vi "Generate New Filename.vi"(8 "Filename Suffix (_data.csv)":string="_data.csv", 9 "Time Format String\n(%y_%m_%d__%H_%M_%S%4u)":string="%y_%m_%d__%H_%M_%S%4u", 10 "Output Directory":path=path "C:/Users/Josh/Desktop/code/CVB/Config/generated_data", 11 "Create New File":bool) -> (3 "Output Filename":path)   [LabVIEW 2021]
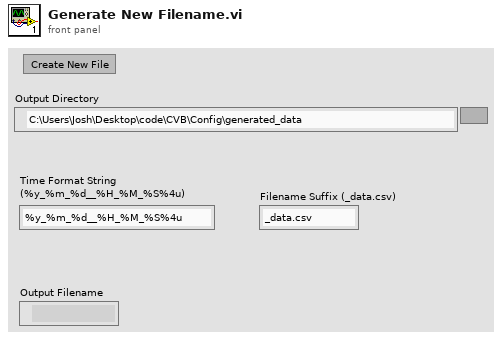
[diagram p1: front panel]
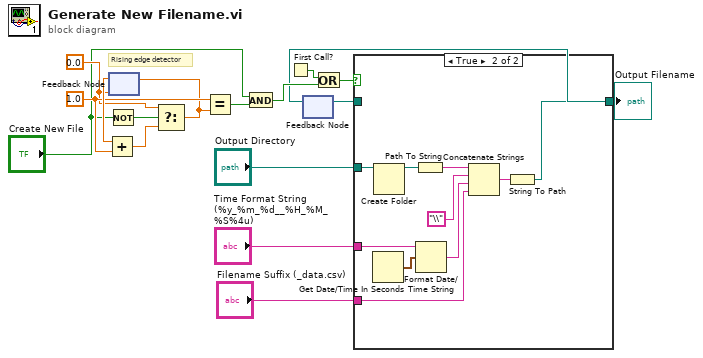
[diagram p0: block diagram]
diagram:
  w12 = 0.0
  w15 = 1.0 ("y")
  # "Rising edge detector"
  n1 = Not(x="Create New File") -> (.not. x?=w10:bool)
  n2 = feedback #1(w12) -> (w16:dbl)
  n3 = Add(x=w16, y=w15) -> (x+y=w11:dbl)
  n4 = Select(t=w12, s=w10, f=w11) -> (s? t:f=w13:dbl)
  n5 = feedback-in #1(w13) -> ()
  n6 = Equal?(x=w15, y=w13) -> (x = y?=w14:bool)
  n7 = And(x="Create New File", y=w14) -> (x .and. y?=w8:bool)
  n8 = First Call?() -> (First Call?: T/F=w7:bool)
  n9 = feedback #2() -> (w6:path)  [unwired: 1 in]
  n10 = Or(x=w7, y=w8) -> (x .or. y?=w9:bool)
  n11 = case shown="True" w9 {
    tunnel: [w17 w20] -> w5
    tunnel: w6 -> [w17 _]
    tunnel: "Output Directory" -> [_ w19]
    tunnel: "Time Format String\n(%y_%m_%d__%H_%M_%S%4u)" -> [_ w22]
    tunnel: "Filename Suffix (_data.csv)" -> [_ w21]
    frame False {
    }
    frame True {
      n12 = Get Date/Time In Seconds() -> (seconds since 1Jan1904=w23:timestamp)
      n13 = Create Folder(path (use dialog)=w19) -> (created path=w18:path)  [unwired: 2 in, 2 out]
      n14 = Path To String(path=w18) -> (string=w26:string)
      n15 = Format Date/Time String(time format string (%c)=w22, seconds (now)=w23) -> (date/time string=w25:string)  [unwired: 1 in]
      n16 = Concatenate Strings(w26, "\\" ("string"), w25, w21) -> (w24:string)
      n17 = String To Path(string=w24) -> (path=w20:path)
    }
  }
  "Output Filename" <- w5
  n18 = feedback-in #2(w5) -> ()
